vi "Add Plugin with Children.vi"(6 "ID":i32, 7 "Plugin Configuration":refnum<class "Plugin Configuration.lvclass">, 8 "error in (no error)":errorcluster, 10 "parent tag":string, 11 "Application Data In":T1={"Item Tree Control"=refnum, "Top-Level VI"=refnum, "menu reference"=refnum, "queue"=refnum, "Stop Pointer"=refnum, "Buffer Variant"=variant, "server ID"=refnum, "framework tag"="", "Values"=refnum, "Hex"=refnum, "ASCII"=refnum, "lines visible"=0, "values padding"=0, "current buffer data"={"decimation"=0, "avg bandwidth"=0.0, "channels"=[], "byte order"=enum."little-endian", "buffer descriptor"={"buffer type"=enum."Engine", "plugin id"=0, "group id"=0, "transfer id"=0, "offset"=0, "length"=0}, "values channels"={"index"=0, "count"=0, "engine offset"=0}, "select start offset"=18446744073709551615, "select end offset"=0, "channel index"=-1}, "Framework Configuration"=refnum} {"current buffer data"."channels"."configuration"."string offset" format="%d bytes"; "current buffer data"."avg bandwidth" format="%.0g bytes"}) -> (0 "error out":errorcluster, 2 "average bandwidth":dbl, 3 "Application Data Out":T1={"Item Tree Control"=refnum, "Top-Level VI"=refnum, "menu reference"=refnum, "queue"=refnum, "Stop Pointer"=refnum, "Buffer Variant"=variant, "server ID"=refnum, "framework tag"="", "Values"=refnum, "Hex"=refnum, "ASCII"=refnum, "lines visible"=0, "values padding"=0, "current buffer data"={"decimation"=0, "avg bandwidth"=0.0, "channels"=[], "byte order"=enum."little-endian", "buffer descriptor"={"buffer type"=enum."Engine", "plugin id"=0, "group id"=0, "transfer id"=0, "offset"=0, "length"=0}, "values channels"={"index"=0, "count"=0, "engine offset"=0}, "select start offset"=18446744073709551615, "select end offset"=0, "channel index"=-1}, "Framework Configuration"=refnum} {"current buffer data"."channels"."configuration"."string offset" format="%d bytes"; "current buffer data"."avg bandwidth" format="%.0g bytes"})   [LabVIEW 2021, in "DSF Core.lvlib"]
uses:
  DSF Core.lvlib
  Main VI/Application Data.ctl
  <vilib>/NI/Memory Manager/Classes/Pointer/Pointer.lvclass
  Classes/Configuration/Core/Framework/Framework Configuration.lvclass
  Buffer Reader/Queue Data.ctl
  Buffer Reader/Buffer Data.ctl
  Classes/Configuration/Core/Transfer/Channel Configuration.ctl
  Typedefs/Core Channel Configuration.ctl
  Typedefs/DSF Data Type.ctl
  Typedefs/DSF Settings Info.ctl
  Typedefs/DSF Byte Order.ctl
  Classes/Thread/Data Server/DSF Buffer Subset Descriptor.ctl
  Typedefs/DSF Buffer Type.ctl
  Main VI/Values Channels.ctl
  Classes/Configuration/Core/Plugin/Plugin Configuration.lvclass
  ID to Tree Items/Tree Item Type.ctl
  Classes/Configuration/Core/Group/Group Configuration.lvclass
  Classes/Configuration/Core/Channel/Channel Configuration.lvclass
  Classes/Configuration/Core/Thread/Thread Configuration.lvclass
  Classes/Configuration/Core/Transfer/Transfer Configuration.lvclass
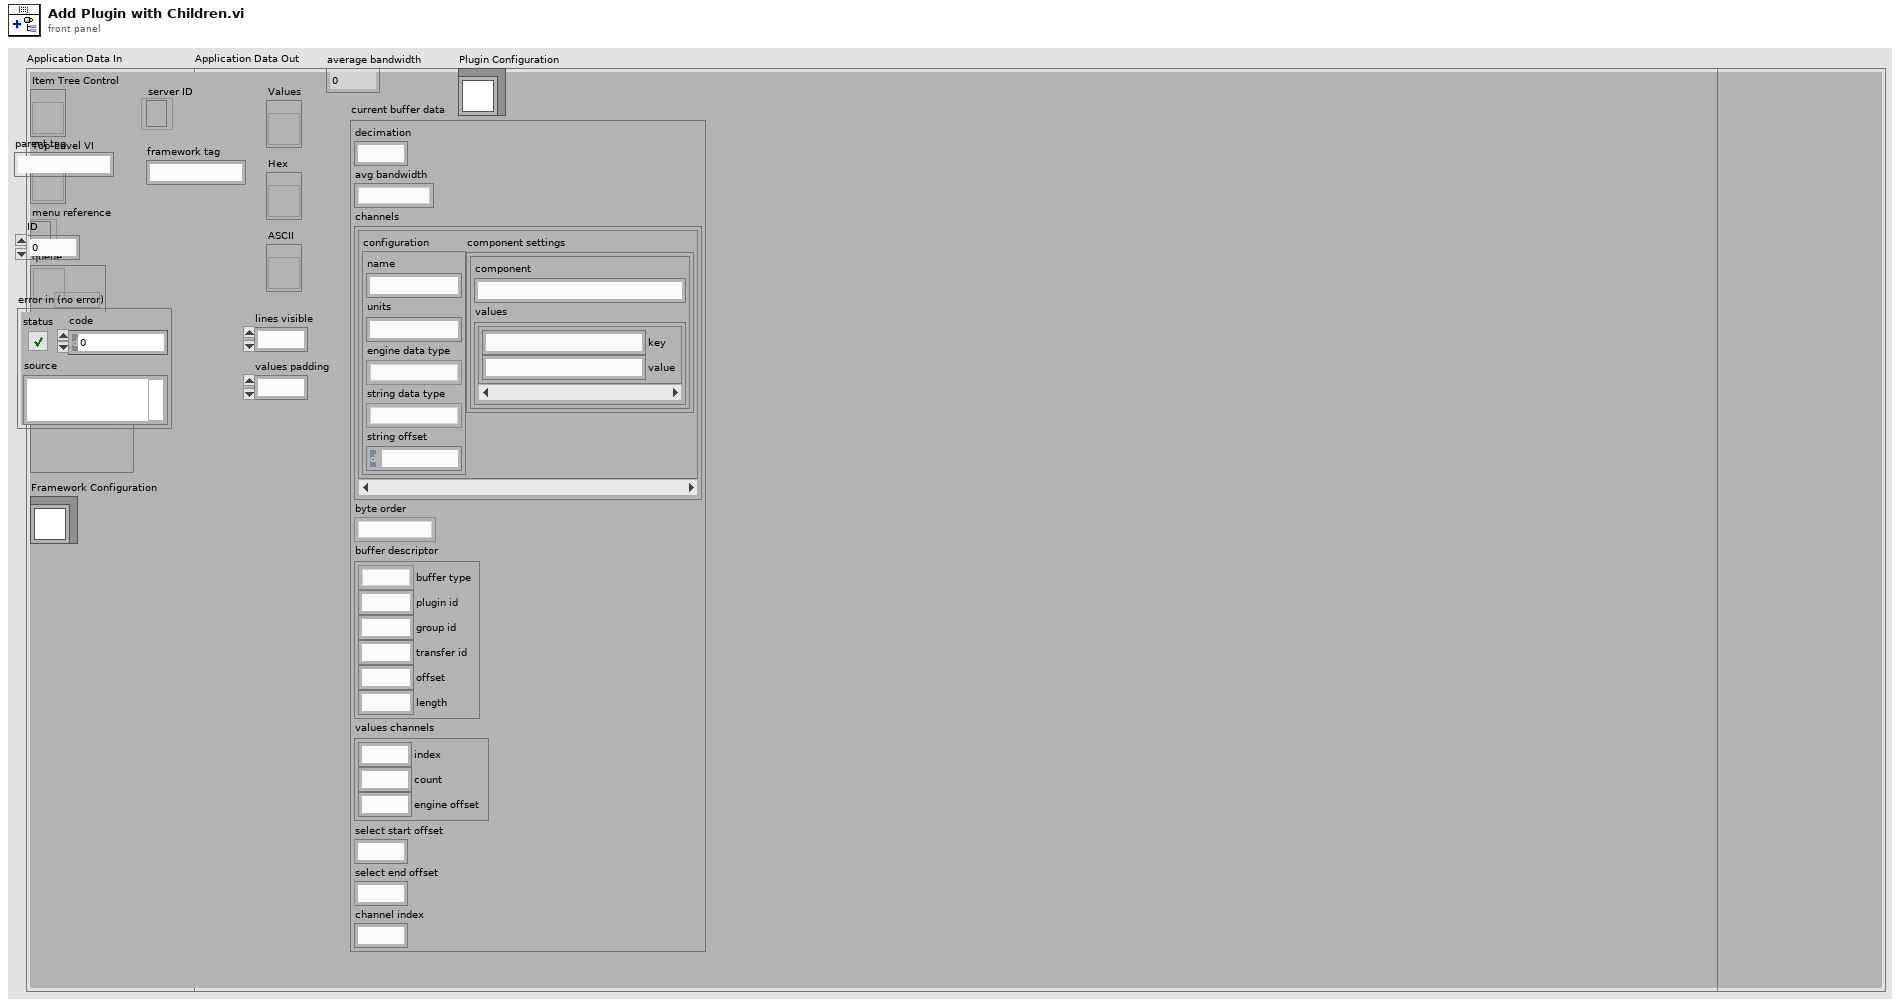
[diagram p1: front panel]
types:
  T1 = typedef "DSF Core.lvlib/Application Data.ctl" = cluster{"Item Tree Control":refnum<vi>, "Top-Level VI":refnum<vi>, "menu reference":refnum<k9>, "queue":refnum<queue>, "Stop Pointer":refnum<class "Pointer.lvclass">, "Buffer Variant":variant, "server ID":refnum<k5>, "framework tag":string, "Values":refnum<vi>, "Hex":refnum<vi>, "ASCII":refnum<vi>, "lines visible":i32, "values padding":i32, "current buffer data":T2, "Framework Configuration":refnum<class "Framework Configuration.lvclass">}
  T2 = typedef "DSF Core.lvlib/Buffer Data.ctl" = cluster{"decimation":u64, "avg bandwidth":dbl, "channels":T3[], "byte order":T7, "buffer descriptor":T8, "values channels":T10, "select start offset":u64, "select end offset":u64, "channel index":i32}
  T3 = typedef "DSF Core.lvlib/Transfer Configuration.lvclass/Channel Configuration.ctl" = cluster{"configuration":T4, "component settings":T6[]}
  T4 = typedef "DSF Core.lvlib/Channel Configuration.lvclass/Core Channel Configuration.ctl" = cluster{"name":string, "units":string, "engine data type":T5, "string data type":T5, "string offset":u64}
  T5 = typedef "DSF Core.lvlib/DSF Data Type.ctl" = enum8{"Bool", "SGL", "DBL", "I8", "I16", "I32", "I64", "U8", "U16", "U32", "U64"}
  T6 = typedef "DSF Core.lvlib/DSF Settings Info.ctl" = cluster{"component":string, "values":cluster{"key":string, "value":string}[]}
  T7 = typedef "DSF Core.lvlib/DSF Byte Order.ctl" = enum8{"big-endian", "little-endian"}
  T8 = typedef "DSF Core.lvlib/DSF Buffer Subset Descriptor.ctl" = cluster{"buffer type":T9, "plugin id":i32, "group id":i32, "transfer id":i32, "offset":u64, "length":i64}
  T9 = typedef "DSF Core.lvlib/DSF Buffer Type.ctl" = enum16{"Engine", "String"}
  T10 = typedef "DSF Core.lvlib/Values Channels.ctl" = cluster{"index":i32, "count":i32, "engine offset":u64}
  T11 = typedef "DSF Core.lvlib/Tree Item Type.ctl" = enum16{"Framework", "Plugin Group", "Plugin", "Group", "Transfer", "Buffer", "Channel"}
  T12 = typedef "DSF Core.lvlib/Plugin Configuration.lvclass/Core Plugin Configuration.ctl" = cluster{"name":string, "components":string[], "cycle timing":T13}
  T13 = typedef "DSF Core.lvlib/DSF Timing Info.ctl" = cluster{"priority":u64, "decimation":u64, "offset":u64}
  T14 = typedef "DSF Core.lvlib/Tree Item.ctl" = cluster{"Left Cell String":string, "Child Text":string[], "Child Tag":string, "Glyph Index":i32}
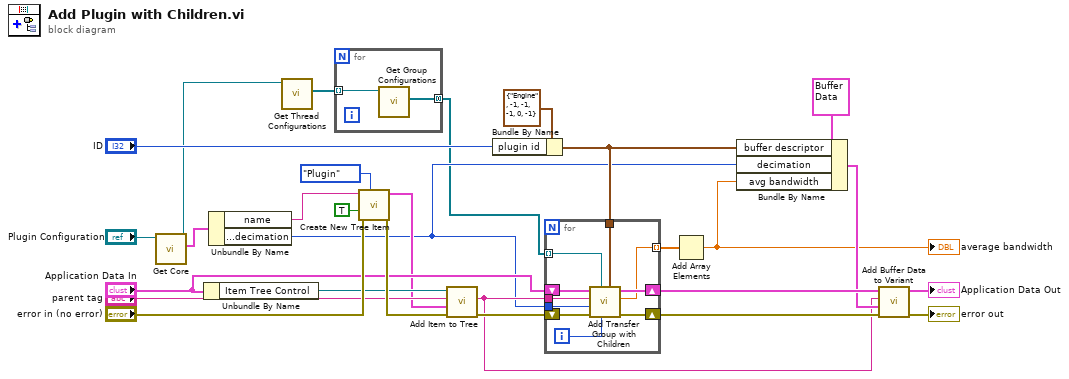
[diagram p0: block diagram]
diagram:
  n1 = call "Get Core.vi"("Plugin Configuration in"="Plugin Configuration") -> ("core"=w3:T12, "Plugin Configuration out"=w2:refnum<class "Plugin Configuration.lvclass">)  [unwired: 8 in, 1 out]
  n2 = Unbundle By Name("Application Data In") -> ("Item Tree Control"=w17:refnum<vi>)
  n3 = Unbundle By Name(w3) -> ("name"=w1:string, "cycle timing.decimation"=w7:u64)
  n4 = call "Get Thread Configurations.vi"("Plugin Configuration in"=w2) -> ("Thread Configurations"=w6:refnum<class "Thread Configuration.lvclass">[])  [unwired: 8 in, 2 out]
  n5 = for {
    tunnel: w6 -> [w30] mode=indexing
    tunnel: [w29] -> w5 mode=concatenating
    n6 = call "Get Group Configurations.vi"("Thread Configuration in"=w30) -> ("Group Configurations"=w29:refnum<class "Group Configuration.lvclass">[])  [unwired: 8 in, 2 out]
  }
  n7 = call "Create New Tree Item.vi"("Item Type"=Tree_Item_Type."Plugin", "error in"="error in (no error)", "found?"=TRUE, "Left Cell String"=w1) -> ("error out"=w28:errorcluster, "Item"=w12:T14)  [unwired: 6 in]
  n8 = call "Add Item to Tree.vi"("error in (no error)"=w28, "Item"=w12, "parent tag"="parent tag", "TreeControl in"=w17) -> ("error out"=w15:errorcluster, "new item tag"=w11:string)  [unwired: 5 in, 1 out]
  n9 = Bundle By Name(cluster=T8 {"buffer type"=enum."Engine", "plugin id"=-1, "group id"=-1, "transfer id"=-1, "offset"=0, "length"=-1} ("buffer descriptor"), "plugin id"="ID") -> (w8:T8)
  n10 = for {
    tunnel: w11 -> [w35]
    tunnel: w7 -> [w36]
    shift-right: [w37] -> w23
    shift-left: "Application Data In" -> [w40]
    shift-right: [w38] -> w22
    shift-left: w15 -> [w39]
    tunnel: [w34] -> w16 mode=indexing
    tunnel: w5 -> [w33] mode=indexing
    tunnel: w8 -> [w31]
    i -> [w32]
    # "Inline Tx Groups"
    n11 = call "Add Transfer Group with Children.vi"("buffer descriptor"=w31, "ID"=w32, "Group Configuration"=w33, "error in (no error)"=w39, "Plugin Decimation (1)"=w36, "parent tag"=w35, "Application Data In"=w40) -> ("error out"=w38:errorcluster, "average bandwidth"=w34:dbl, "Application Data In"=w37:T1)  [unwired: 2 in]
  }
  n12 = Add Array Elements(numeric array=w16) -> (sum=w13:dbl)
  "average bandwidth" <- w13
  n13 = Bundle By Name(cluster=T2 {"decimation"=0, "avg bandwidth"=0.0, "channels"=[], "byte order"=enum."big-endian", "buffer descriptor"={"buffer type"=enum."Engine", "plugin id"=0, "group id"=0, "transfer id"=0, "offset"=0, "length"=0}, "values channels"={"index"=0, "count"=0, "engine offset"=0}, "select start offset"=18446744073709551615, "select end offset"=0, "channel index"=-1} ("Buffer data"), "buffer descriptor"=w8, "decimation"=w7, "avg bandwidth"=w13) -> (w14:T2)
  n14 = call "Add Buffer Data to Variant.vi"("error in (no error)"=w22, "Buffer data"=w14, "tag"=w11, "Application Data In in"=w23) -> ("error out"=→"error out":errorcluster, "Application Data In out"=→"Application Data Out":T1)  [unwired: 6 in]
